vi "RT_Velocity mode_Oct19.vi"() -> ()   [LabVIEW 2018]
uses:
  <vilib>/Platform/TimedLoop/XDataNode/timing_clust.ctl
  <vilib>/Platform/TimedLoop/XDataNode/nitl_modes.ctl
  <vilib>/Platform/TimedLoop/XDataNode/wakeup.ctl
  <vilib>/Analysis/baseanly.llb/Mean (DBL).vi
  <vilib>/FPGAPlugInAG/myRIO-1900/niLvFpga_Open_myRIO-1900.vi
  <vilib>/rvi/interface/common/dynamic/niFpgaDynamicAddResources.vi
  <vilib>/Utility/error.llb/Error Cluster From Error Code.vi
  <vilib>/rvi/errors/niLvFpgaAdjustHostInterfaceError.vi
  <vilib>/FPGAPlugInAG/Dynamic/niLvFpga_Close_Dynamic.vi
  <vilib>/rvi/interface/nirviOpenFPGA/nirviOpenFPGA.xnode
  UNCC Watt balance Oct19/FPGA Bitfiles/UNCCWattbalanceO_FPGATarget_fpgaW&RADCW2DACs_bUgWeZ5fmbw.lvbitx
  FPGA files/fpga_W&R_ADC_W_2DACs_Write_then_CLK.vi
  <vilib>/Platform/TimedLoop/XDataNode/XDataNode.xnode
  <vilib>/rvi/interface/nirviReadWriteControl/nirviReadWriteControl.xnode
  <vilib>/rvi/interface/nirviCloseFPGA/nirviCloseFPGA.xnode
  <vilib>/Platform/TimedLoop/XDataNode/XDNodeRunTimeDep.lvlib
  NiFpgaLv.dll
  <vilib>/rvi/interface/Simulation/niFpgaSimulationCallBeginRW.vi
  <vilib>/Analysis/NI_AALBase.lvlib
panel:
  out "EMF 2":cluster{dbl, dbl}(graph)={0.4520936579705314, 0.027144971542792554}
  out "min velocity":dbl=-0.04070982803607118 format="%^#_6e"
  out "max velocity":dbl=0.04911729252178159 format="%^#_6e"
  out "min EMF":dbl=-0.4868518495573308 format="%^#_6e"
  out "max EMF":dbl=0.6606955113451366 format="%^#_6e"
  out "BL (avg.)":dbl(graph)=11.501948675236207
  in  "Gain":dbl=5.7903
  in  "init Max array":i32=500
  out "EMF":dbl(graph)=0.4520936579705314
  out "velocity":dbl(graph)=0.030272975571051484
  in  "pos on/off":bool=TRUE
  out "Displacement (m)":dbl(graph)=-0.00013937928193234351
  out "init array_moving avg. EMF":dbl[](array[numeric])
  out "no. moving avg. EMF":u8=1
  out "init array_moving avg. Z":dbl[](array[numeric])
  in  "no. moving avg. Z":u8=1
  in  "CH1":bool[](array[boolean])=[FALSE, FALSE, FALSE, FALSE, FALSE, TRUE, FALSE, FALSE, FALSE, FALSE, FALSE, FALSE, FALSE, FALSE, FALSE, FALSE]
  in  "CH3":bool[](array[boolean])=[FALSE, FALSE, TRUE, FALSE, FALSE, FALSE, FALSE, FALSE, FALSE, FALSE, FALSE, FALSE, FALSE, FALSE, FALSE, FALSE]
  in  "offset (mV)":dbl
  in  "amplitude (V)":dbl=0.9
  in  "frequency (Hz)":dbl=25.0
  out "avg loop rate":dbl=3.943982652692447
  in  "Stop Button":bool
  in  "delay (us)":u32=250
  out "Finished Late? [i-1]":bool
  # "+/- 10 V range"
  # "+/- 5 V range"
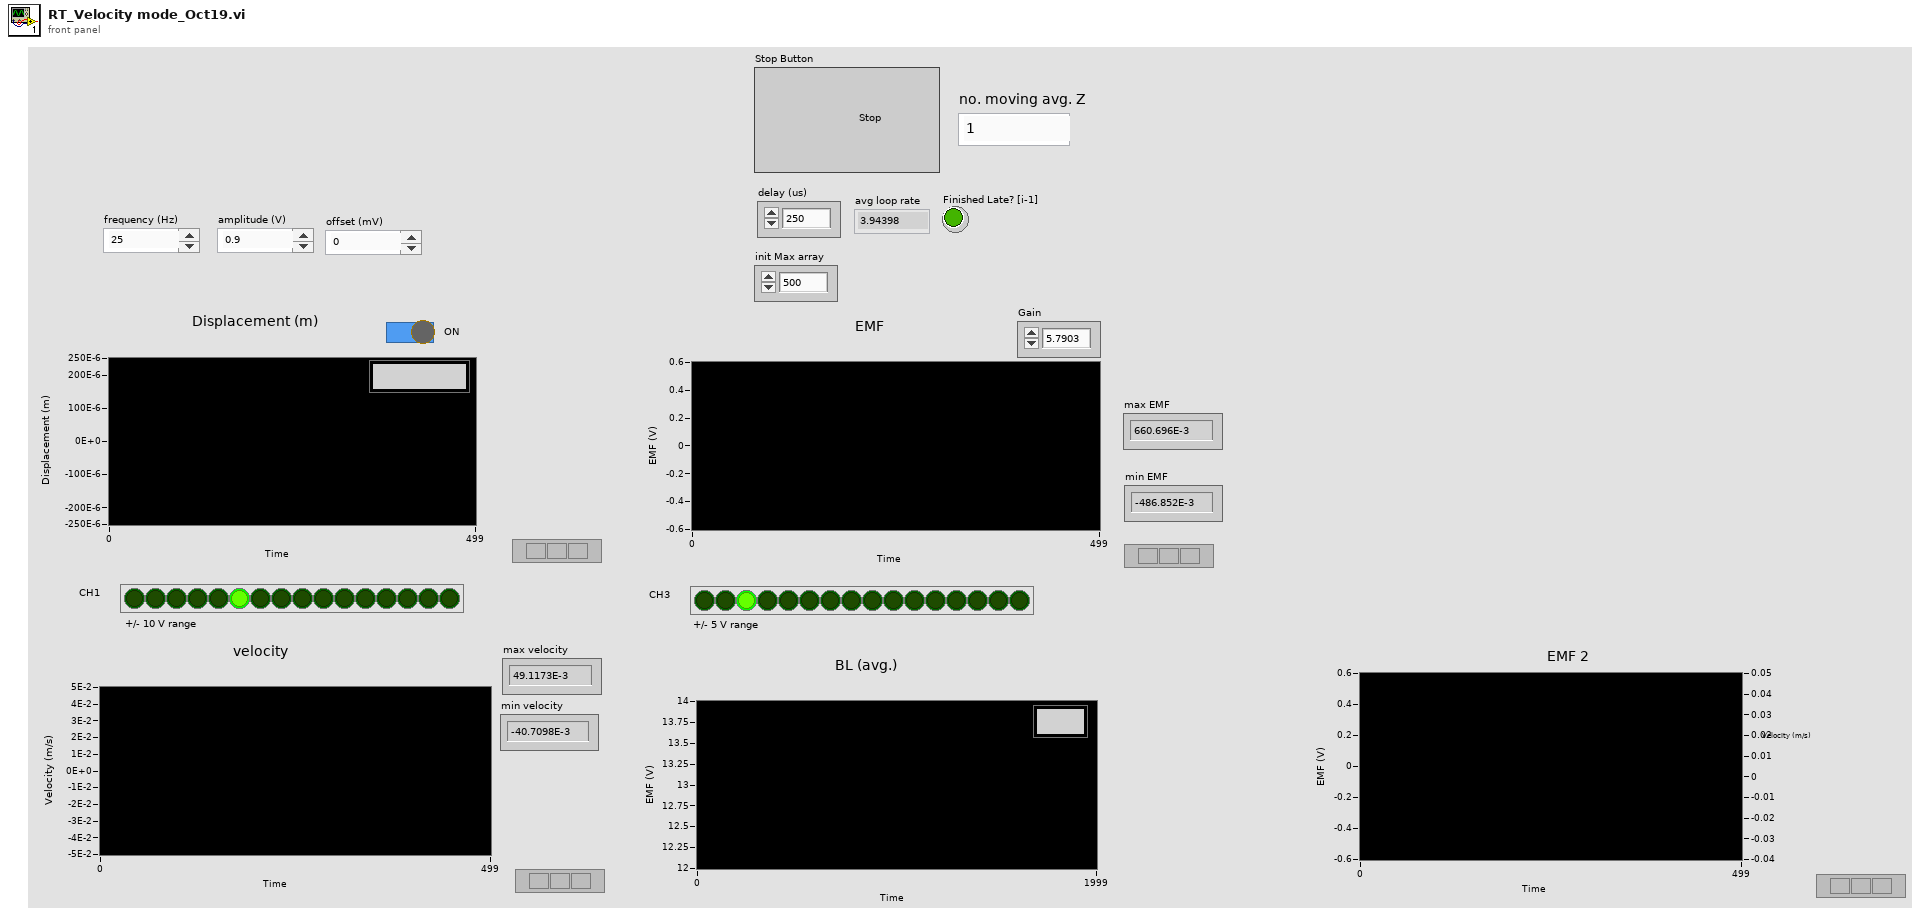
[diagram p1: front panel]
types:
  T1 = typedef "XDNodeRunTimeDep.lvlib/timing_clust.ctl" = cluster{"Expected End [f-1]":u64, "Actual End [f-1]":u64, "Finished Late? [f-1]":bool, "Expected End [i-1]":u64, "Actual End [i-1]":u64, "Finished Late? [i-1]":bool, "Expected Start [i]":u64, "Actual Start [i]":u64, "Expected Start [f]":u64, "Actual Start [f]":u64, "Source Name":string, "Structure Name":string, "Period":i64, "Deadline":i64, "Offset":i64, "Start":i64, "Priority":i32, "Timeout":i32, "Mode":T2, "Wakeup Reason":T3, "Error":errorcluster, "Source Type":string, "Secondary Source Type":string, "Global End Time":u64, "Global Start Time":u64, "Frame Duration":u64, "Iteration Duration":u64, "Assigned CPU":i32, "I/O Scan Engine Mode":u32}
  T2 = typedef "XDNodeRunTimeDep.lvlib/nitl_modes.ctl" = enum32{"No Change", "Process missed periods, maintain original phase", "Discard missed periods, maintain original phase", "Process missed periods, ignore original phase", "Discard missed periods, ignore original phase"}
  T3 = typedef "XDNodeRunTimeDep.lvlib/wakeup.ctl" = enum32{"Normal", "Aborted", "Asynchronous wakeup", "Timing source error", "Timed loop error", "Timeout"}
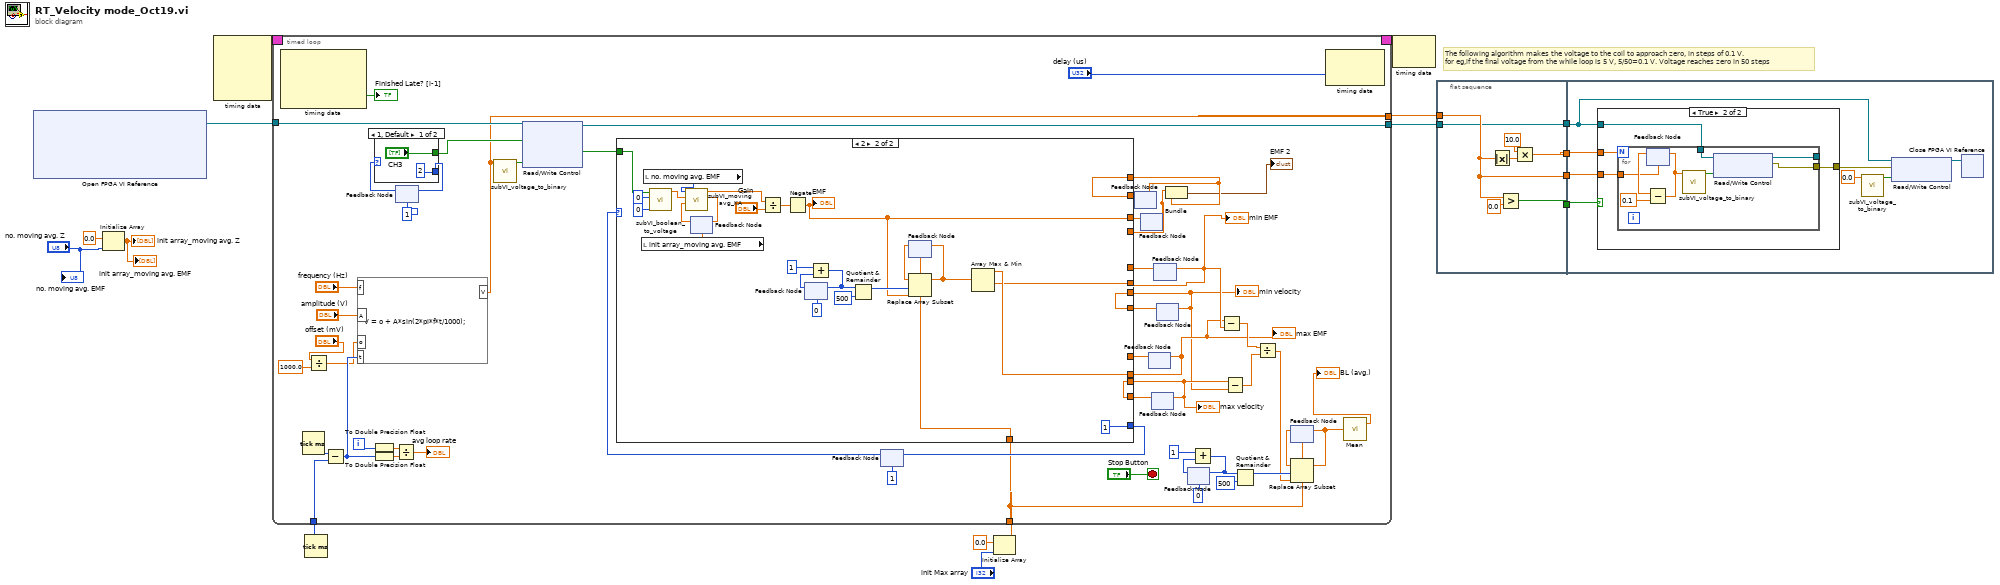
[diagram p0: block diagram]
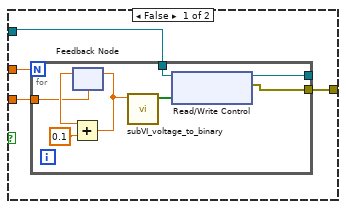
[diagram p2: hidden frame]
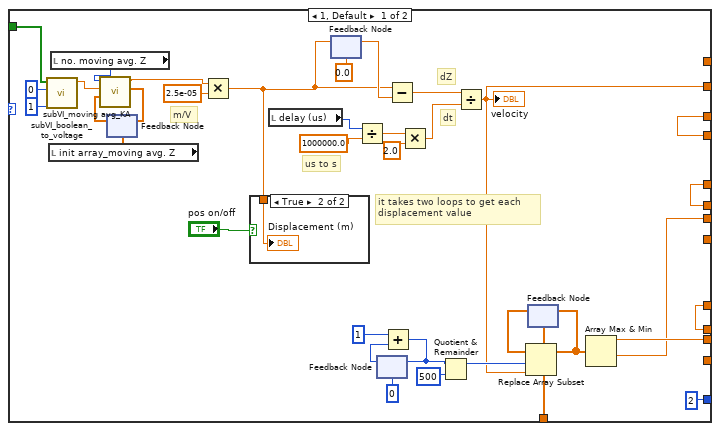
[diagram p3: hidden frame]
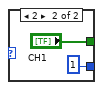
[diagram p5: hidden frame]
diagram:
  # "The following algorithm makes the voltage to the coil to approach zero, in steps of 0.1 V.\nfor eg,if the final voltage from the while loop is 5 V, 5/50=0.1 V. Voltage reaches zero in 50 steps"
  n1 = xnode "Open FPGA VI Reference"() -> ("FPGA VI Reference Out"=w14:refnum<k20>)  [unwired: 2 in, 1 out]
  n2 = Initialize Array(0.0 ("element"), "no. moving avg. Z") -> (→"init array_moving avg. Z" →"init array_moving avg. EMF":dbl[])
  n3 = node-c288() -> (w16:T1)  [unwired: 4 in]
  n4 = Tick Count (ms)() -> (millisecond timer value=w13:u32)
  n5 = Initialize Array(0.0 ("element"), "init Max array") -> (w7:dbl[])
  n6 = timed-loop {
    tunnel: w14 -> [w69]
    timing: w16 -> [_]
    timing-out: [_] -> w15
    tunnel: [w59] -> w1
    tunnel: w13 -> [w54]
    tunnel: w7 -> [w41]
    tunnel: [w18] -> w3
    i -> [w53]
    stop <- "Stop Button" stop-if-true
    n7 = node-c288() -> (→"Finished Late? [i-1]":bool)  [unwired: 1 in, 3 out]
    n8 = Tick Count (ms)() -> (millisecond timer value=w58:u32)
    n9 = Divide(x="offset (mV)", y=1000.0) -> (x/y=w28:dbl)
    n10 = Subtract(x=w58, y=w54) -> (x-y=w48:u32)
    n11 = formula code="V = o + A*sin(2*pi*f*t/1000);"("f"="frequency (Hz)", "A"="amplitude (V)", "t"=w48, "o"=w28) -> ("V"=w18:dbl)
    n12 = To Double Precision Float(number=w53) -> (double precision float=w56:dbl)
    n13 = To Double Precision Float(number=w48) -> (double precision float=w57:dbl)
    n14 = Divide(x=w56, y=w57) -> (x/y=→"avg loop rate":dbl)
    n15 = feedback #1(1) -> (w67:i32)
    n16 = case shown="1, Default" w67 {
      tunnel: ["CH3" "CH1"] -> w50
      tunnel: [2 1] -> w65
      frame 1, Default {
      }
      frame 2 {
      }
    }
    n17 = feedback-in #1(w65) -> ()
    n18 = call "subVI_voltage_to_binary.vi"("voltage"=w18) -> ("binary"=w49:bool[])  [unwired: 10 in]
    n19 = xnode "Read/Write Control"("FPGA VI Reference In"=w69, "ADC write"=w50, "DAC 1 write"=w49) -> ("FPGA VI Reference Out"=w59:refnum<k20>, "ADC read"=w17:bool[])  [unwired: 1 in, 1 out]
    n20 = feedback #2(1) -> (w64:i32)
    n21 = feedback #3() -> (w20:dbl)  [unwired: 1 in]
    n22 = feedback #4() -> (w22:dbl)  [unwired: 1 in]
    n23 = feedback #5() -> (w47:dbl)  [unwired: 1 in]
    n24 = feedback #6() -> (w46:dbl)  [unwired: 1 in]
    n25 = feedback #7() -> (w34:dbl)  [unwired: 1 in]
    n26 = feedback #8() -> (w35:dbl)  [unwired: 1 in]
    n27 = case shown="2" w64 {
      tunnel: [2 1] -> w62
      tunnel: w41 -> [w88 w125]
      tunnel: [w84 w124] -> w25
      tunnel: [w86 w121] -> w26
      tunnel: w47 -> [w86 _]
      tunnel: w46 -> [_ w124]
      tunnel: [w85 w120] -> w27
      tunnel: [w83 w119] -> w24
      tunnel: w35 -> [_ w119]
      tunnel: w34 -> [w85 _]
      tunnel: [w81 w118] -> w21
      tunnel: [w82 w116] -> w23
      tunnel: w22 -> [w82 _]
      tunnel: w20 -> [_ w118]
      tunnel: w17 -> [w78 w113]
      frame 1, Default {
        # "dZ"
        # "dt"
        # "us to s"
        # "it takes two loops to get each displacement value"
        # "m/V"
        n28 = call "subVI_boolean_to_voltage.vi"("Gain"=i16 1, "UNI"=i16 0, "ADC read"=w78) -> ("V"=w79:dbl)  [unwired: 8 in]
        n29 = local read "init array_moving avg. Z"() -> (w106:dbl[])
        n30 = local read "no. moving avg. Z"() -> (w109:u8)
        n31 = feedback #9(w106) -> (w108:dbl[])
        n32 = call "subVI_moving avg_KA.vi"("input array"=w108, "sample"=w79, "no. moving avg."=w109) -> ("output array"=w107:dbl[], "avg."=w80:dbl)  [unwired: 7 in]
        n33 = feedback-in #9(w107) -> ()
        n34 = Multiply(x=w80, y=2.5e-05) -> (x*y=w75:dbl)
        n35 = case shown="True" "pos on/off" {
          tunnel: w75 -> [_ w111]
          frame False {
          }
          frame True {
            "Displacement (m)" <- w111
          }
        }
        n36 = local read "delay (us)"() -> (w96:u32)
        n37 = feedback #10(0.0) -> (w97:dbl)
        n38 = feedback-in #10(w75) -> ()
        n39 = Divide(x=w96, y=1000000.0) -> (x/y=w102:dbl)
        n40 = feedback #11(u16 0) -> (w95:u16)
        n41 = Add(x=u16 1, y=w95) -> (x+y=w92:u16)
        n42 = feedback-in #11(w92) -> ()
        n43 = Subtract(x=w75, y=w97) -> (x-y=w99:dbl)
        n44 = Multiply(x=w102, y=2.0 ("x")) -> (x*y=w103:dbl)
        n45 = Quotient & Remainder(x=w92, y=u16 500) -> (x-y*floor(x/y)=w90:u16)  [unwired: 1 out]
        n46 = Divide(x=w99, y=w103) -> (x/y=w81:dbl)
        "velocity" <- w81
        n47 = feedback #12(w88) -> (w89:dbl[])
        n48 = Replace Array Subset(array=w89, new element=w81, index=w90) -> (w87:dbl[])
        n49 = feedback-in #12(w87) -> ()
        n50 = Array Max & Min(array=w87) -> (max value=w84:dbl, min value=w83:dbl)  [unwired: 2 out]
      }
      frame 2 {
        n51 = local read "init array_moving avg. EMF"() -> (w137:dbl[])
        n52 = local read "no. moving avg. EMF"() -> (w134:u8)
        n53 = call "subVI_boolean_to_voltage.vi"("Gain"=i16 0, "UNI"=i16 0, "ADC read"=w113) -> ("V"=w112:dbl)  [unwired: 8 in]
        n54 = feedback #13(w137) -> (w135:dbl[])
        n55 = call "subVI_moving avg_KA.vi"("input array"=w135, "sample"=w112, "no. moving avg."=w134) -> ("output array"=w136:dbl[], "avg."=w123:dbl)  [unwired: 7 in]
        n56 = feedback-in #13(w136) -> ()
        n57 = Divide(x=w123, y="Gain") -> (x/y=w117:dbl)
        n58 = Negate(x=w117) -> (-x=w116:dbl)
        "EMF" <- w116
        n59 = feedback #14(u16 0) -> (w133:u16)
        n60 = Add(x=u16 1, y=w133) -> (x+y=w130:u16)
        n61 = feedback-in #14(w130) -> ()
        n62 = Quotient & Remainder(x=w130, y=u16 500) -> (x-y*floor(x/y)=w128:u16)  [unwired: 1 out]
        n63 = feedback #15(w125) -> (w126:dbl[])
        n64 = Replace Array Subset(array=w126, new element=w116, index=w128) -> (w127:dbl[])
        n65 = feedback-in #15(w127) -> ()
        n66 = Array Max & Min(array=w127) -> (max value=w121:dbl, min value=w120:dbl)  [unwired: 2 out]
      }
    }
    "max velocity" <- w25
    "min velocity" <- w24
    "max EMF" <- w26
    "min EMF" <- w27
    n67 = feedback-in #2(w62) -> ()
    n68 = feedback-in #3(w21) -> ()
    n69 = feedback-in #4(w23) -> ()
    n70 = feedback-in #5(w26) -> ()
    n71 = feedback-in #6(w25) -> ()
    n72 = feedback-in #7(w27) -> ()
    n73 = feedback-in #8(w24) -> ()
    n74 = Bundle(w22, w20) -> (→"EMF 2":cluster{dbl, dbl})  [unwired: 1 in]
    n75 = feedback #16(u16 0) -> (w45:u16)
    n76 = Add(x=u16 1, y=w45) -> (x+y=w43:u16)
    n77 = feedback-in #16(w43) -> ()
    n78 = Subtract(x=w26, y=w27) -> (x-y=w33:dbl)
    n79 = Subtract(x=w25, y=w24) -> (x-y=w32:dbl)
    n80 = Quotient & Remainder(x=w43, y=u16 500) -> (x-y*floor(x/y)=w36:u16)  [unwired: 1 out]
    n81 = Divide(x=w33, y=w32) -> (x/y=w31:dbl)
    n82 = feedback #17(w41) -> (w40:dbl[])
    n83 = Replace Array Subset(array=w40, new element=w31, index=w36) -> (w39:dbl[])
    n84 = feedback-in #17(w39) -> ()
    n85 = node-c288("delay (us)") -> ()  [unwired: 1 in, 1 out]
    n86 = call-poly <vilib>:"Mean.vi"("X"=w39) -> ("mean"=→"BL (avg.)":dbl)  [unwired: 1 out]
  }
  n87 = node-c288(w15) -> ()  [unwired: 1 out]
  n88 = flat-sequence {
    tunnel: [w148] -> w6
    tunnel: [w143] -> w5
    tunnel: [w147] -> w4
    tunnel: w3 -> [w147]
    tunnel: [w145] -> w2
    tunnel: w1 -> [w145]
    tunnel: w6 -> [w154]
    tunnel: w5 -> [w152]
    tunnel: w4 -> [w153]
    tunnel: w2 -> [w151]
    frame #0 {
      n89 = Absolute Value(x=w147) -> (abs(x)=w144:dbl)
      n90 = Greater?(x=w147, y=0.0) -> (0:w148:bool)
      n91 = Multiply(x=10.0, y=w144) -> (x*y=w143:dbl)
    }
    frame #1 {
      n92 = case shown="True" w154 {
        tunnel: w152 -> [w161 w173]
        tunnel: w153 -> [w160 w172]
        tunnel: w151 -> [w159 w171]
        tunnel: [w158 w170] -> w150
        frame False {
          n93 = for {
            N: w161 -> [_]
            tunnel: [w168] -> _
            tunnel: w160 -> [w165]
            tunnel: w159 -> [w164]
            tunnel: [w162] -> w158
            n94 = feedback #18(w165) -> (w166:dbl)
            n95 = Add(x=w166, y=0.1) -> (x+y=w163:dbl)
            n96 = feedback-in #18(w163) -> ()
            n97 = call "subVI_voltage_to_binary.vi"("voltage"=w163) -> ("binary"=w169:bool[])  [unwired: 10 in]
            n98 = xnode "Read/Write Control"("FPGA VI Reference In"=w164, "DAC 1 write"=w169) -> ("FPGA VI Reference Out"=w168:refnum<k20>, "error out"=w162:errorcluster)  [unwired: 1 in]
          }
        }
        frame True {
          n99 = for {
            N: w173 -> [_]
            tunnel: [w180] -> _
            tunnel: w172 -> [w177]
            tunnel: w171 -> [w176]
            tunnel: [w174] -> w170
            n100 = feedback #19(w177) -> (w179:dbl)
            n101 = Subtract(x=w179, y=0.1) -> (x-y=w175:dbl)
            n102 = feedback-in #19(w175) -> ()
            n103 = call "subVI_voltage_to_binary.vi"("voltage"=w175) -> ("binary"=w181:bool[])  [unwired: 10 in]
            n104 = xnode "Read/Write Control"("FPGA VI Reference In"=w176, "DAC 1 write"=w181) -> ("FPGA VI Reference Out"=w180:refnum<k20>, "error out"=w174:errorcluster)  [unwired: 1 in]
          }
        }
      }
      n105 = call "subVI_voltage_to_binary.vi"("voltage"=0.0) -> ("binary"=w156:bool[])  [unwired: 10 in]
      n106 = xnode "Read/Write Control"("FPGA VI Reference In"=w151, "error in"=w150, "DAC 1 write"=w156) -> ("FPGA VI Reference Out"=w157:refnum<k20>)  [unwired: 1 out]
      n107 = xnode "Close FPGA VI Reference"("FPGA VI Reference In"=w157) -> ()  [unwired: 1 in, 1 out]
    }
  }
  "no. moving avg. EMF" <- "no. moving avg. Z"
